vi "Prep Controller.vi"(6 "Interlock Q Class":refnum<class "Interlock Q Class.lvclass">, 8 "error in (no error)":errorcluster, 9 "DAQ Data":refnum<data-value>, 10 "Process State Data":refnum<data-value>, 11 "DAQ Controller in":refnum<class "DAQ Controller.lvclass">) -> (0 "error out":errorcluster, 3 "DAQ Controller out":refnum<class "DAQ Controller.lvclass">)   [LabVIEW 2022 SP3, in "DAQ Controller.lvclass"]
uses:
  DAQ Controller.lvclass
  XY Stage/Process Actor/Process Framework/Interlock Q Class/Interlock Q Class.lvclass
  XY Stage/Process Actor/Process Framework/Process State Data/Process State Data.lvclass
  DAQ Data/DAQ Data.lvclass
  DAQ Controller.lvclass/DAQ Controller.ctl
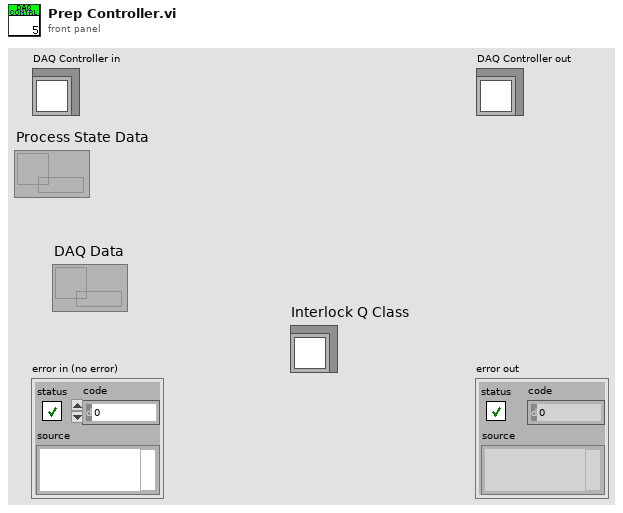
[diagram p1: front panel]
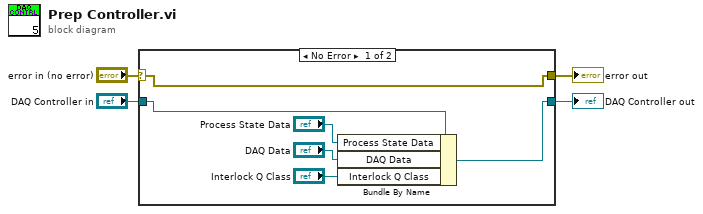
[diagram p0: block diagram]
diagram:
  n1 = case shown="No Error" "error in (no error)" {
    selector: "error in (no error)" -> [w9 w12]
    tunnel: [w9 w12] -> w3
    tunnel: [w8 w11] -> w1
    tunnel: "DAQ Controller in" -> [w10 w11]
    frame No Error {
      n2 = Bundle By Name(cluster=w10, "Process State Data"="Process State Data", "DAQ Data"="DAQ Data", "Interlock Q Class"="Interlock Q Class") -> (w8:refnum<class "DAQ Controller.lvclass">)
    }
    frame Error {
    }
  }
  "error out" <- w3
  "DAQ Controller out" <- w1
